vi "获取阵列信息.vi"(8 "error in (no error)":errorcluster, 11 "MB session in":refnum<class "MB_Master.lvclass">) -> (0 "error out":errorcluster, 2 "阵列信息":cluster{"阵列电压V":dbl, "阵列电流A":dbl, "发电功率W":dbl}, 3 "MB session out":refnum<class "MB_Master.lvclass">)   [LabVIEW 2016, in "采配水.lvlib"]
uses:
  <vilib>/Plasmionique/MB Master/MB_Master/MB_Master.lvclass
  <vilib>/Plasmionique/MB Master/MB Master.lvlib
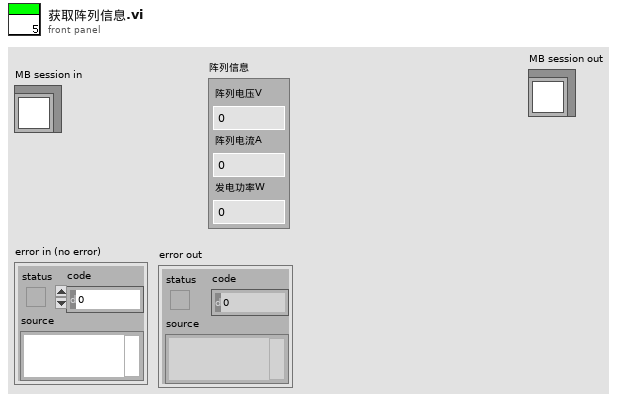
[diagram p1: front panel]
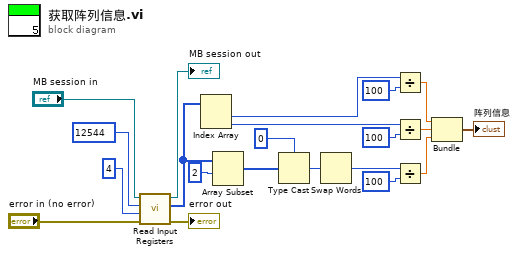
[diagram p0: block diagram]
diagram:
  n1 = call <vilib>:"Read Input Registers.vi"("error in (no error)"="error in (no error)", "quantity"=u16 4, "starting address"=u16 12544, "MB session in"="MB session in") -> ("error out"=→"error out":errorcluster, "Registers"=w17:u16[], "MB session out"=→"MB session out":refnum<class "MB_Master.lvclass">)  [unwired: 5 in]
  n2 = Index Array(array=w17) -> (element #1=w14:u16, element #2=w13:u16)  [unwired: 2 in]
  n3 = Array Subset(array=w17, index=2 ("索引")) -> (w6:u16[])  [unwired: 1 in]
  n4 = Type Cast(type=0, x=w6) -> (*(type *) &x=w4:i32)
  n5 = Swap Words(1:w4) -> (0:w3:i32)
  n6 = Divide(x=w14, y=u16 100) -> (x/y=w10:dbl)
  n7 = Divide(x=w13, y=u16 100) -> (x/y=w9:dbl)
  n8 = Divide(x=w3, y=100) -> (x/y=w8:dbl)
  n9 = Bundle(w10, w9, w8) -> (→"阵列信息":cluster{dbl, dbl, dbl})  [unwired: 1 in]
